vi "Result_Test.vi"(8 "error in (no error)":errorcluster caption="entrée d'erreur (pas d'erreur)", 11 "Delay en entrée":refnum<class "P2056_Provisionning.lvclass">) -> (0 "error out":errorcluster caption="sortie d'erreur", 3 "Delay en sortie":refnum<class "P2056_Provisionning.lvclass">)   [LabVIEW 2020, in "Library Test.lvlib" / "P2056_Provisionning.lvclass"]
uses:
  P2056_Provisionning.lvclass
  C:/Users/ngarcin/OneDrive - Altyor/Standard TB/Class/Test/Test (Default)/Test (Default).lvclass
  Test_Without_Instr/Test_Without_Inst.lvclass
  P2056_Provisionning.lvclass/P2056_Provisionning.ctl
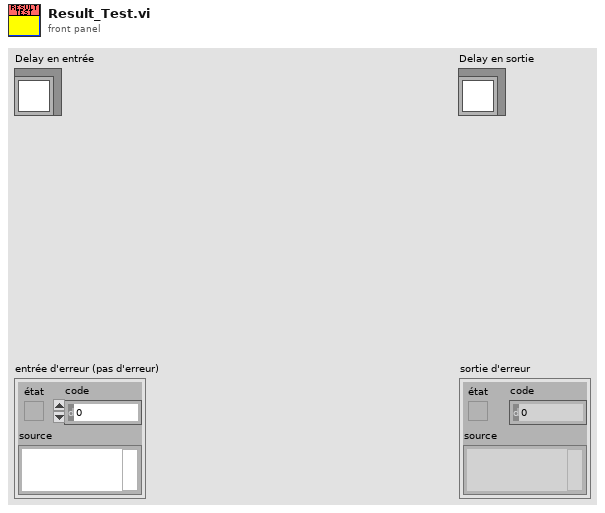
[diagram p1: front panel]
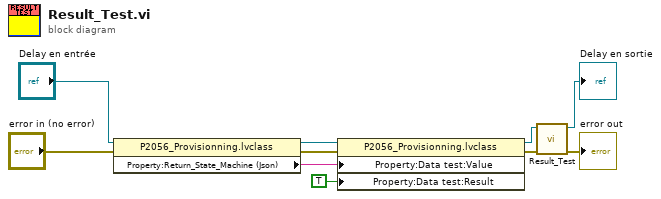
[diagram p0: block diagram]
diagram:
  n1 = property class="P2056_Provisionning.lvclass"(reference="Delay en entrée", error in="error in (no error)") -> (reference out=w7:refnum<class "P2056_Provisionning.lvclass">, error out=w6:errorcluster, "Property:Return_State_Machine (Json)"=w8:string)
  n2 = property class="P2056_Provisionning.lvclass"(reference=w7, error in=w6, "Property:Data test:Value"=w8, "Property:Data test:Result"=TRUE ("Result")) -> (reference out=w2:refnum<class "P2056_Provisionning.lvclass">, error out=w3:errorcluster)
  n3 = call-parent "Result_Test.vi"("error in (no error)"=w3, "Test_Without_Inst en entrée"=w2) -> ("error out"=→"error out":errorcluster, "Test_Without_Inst en sortie"=→"Delay en sortie":refnum<class "P2056_Provisionning.lvclass">)  [unwired: 8 in]
